vi "Generate Error.vi"(8 "error in (no error)":errorcluster, 11 "Sample Error Reporter in":refnum<class "Sample Error Reporter.lvclass">) -> (0 "error out":errorcluster, 3 "Sample Error Reporter out":refnum<class "Sample Error Reporter.lvclass">)   [LabVIEW 2024, in "Sample Error Reporter.lvlib" / "Sample Error Reporter.lvclass"]
uses:
  Sample Error Reporter.lvclass
  Sample Error Reporter.lvclass/Sample Error Reporter.ctl
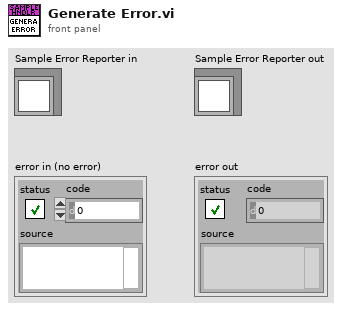
[diagram p1: front panel]
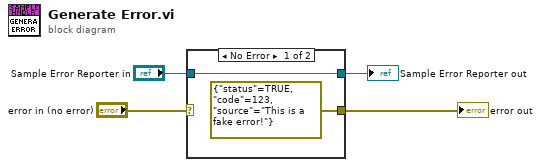
[diagram p0: block diagram]
diagram:
  n1 = case shown="No Error" "error in (no error)" {
    selector: "error in (no error)" -> [_ w8]
    tunnel: [errorcluster {"status"=TRUE, "code"=123, "source"="This is a fake error!"} ("error constant") w8] -> w3
    tunnel: [w6 w7] -> w1
    tunnel: "Sample Error Reporter in" -> [w6 w7]
    frame No Error {
    }
    frame Error {
    }
  }
  "error out" <- w3
  "Sample Error Reporter out" <- w1
